vi "Search_1d_array_element.vi"(6 "error in (no error)":errorcluster, 7 "Count in":string[](array[string]), 8 "BD Date":string[](array[string]), 9 "Elements Found in":string[](array[string])) -> (0 "error out":errorcluster, 1 "Count out":string[](array[string]), 3 "Elements Found out":string[](array[string]))   [LabVIEW 2017]
panel:
  out "Table":string[](array[string])
  # "2020-12-03"
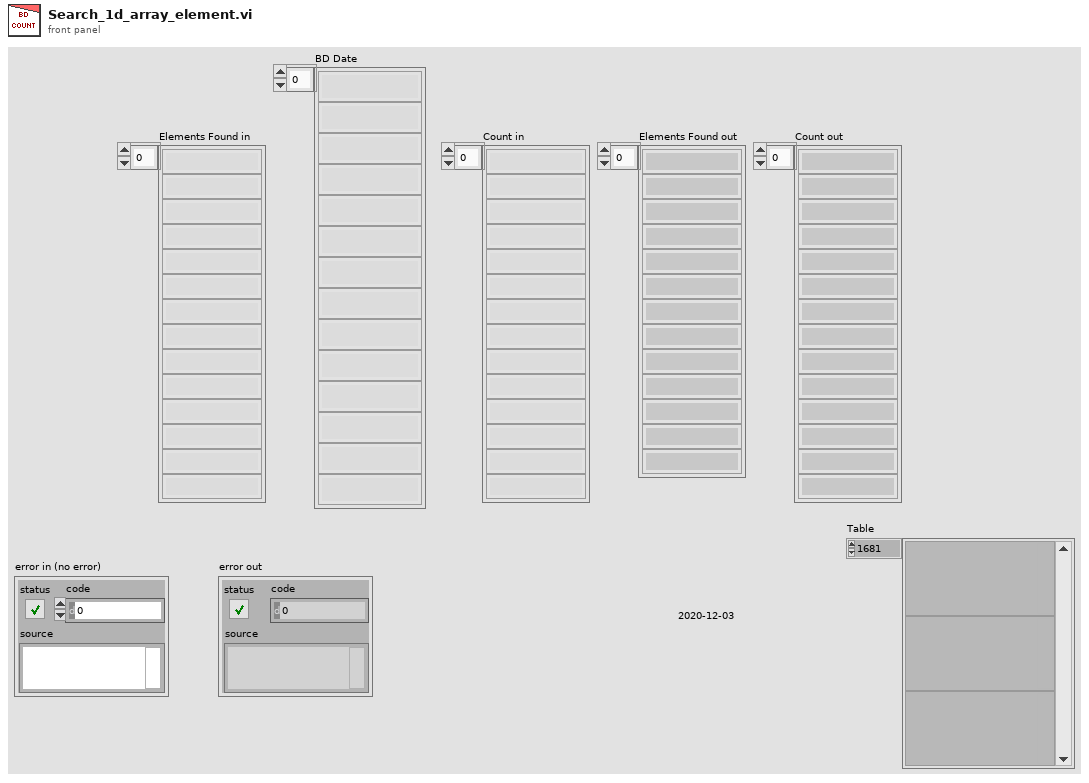
[diagram p1: front panel]
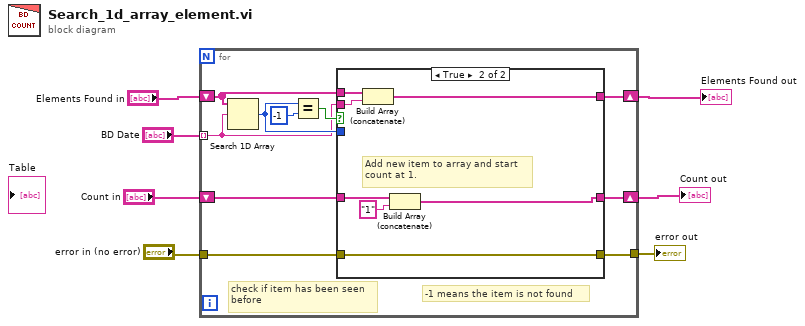
[diagram p0: block diagram]
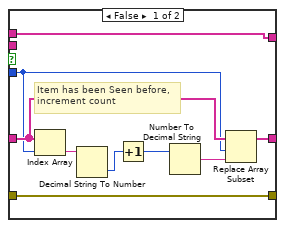
[diagram p2: hidden frame]
diagram:
  n1 = for {
    tunnel: "BD Date" -> [w8] mode=indexing
    shift-right: [w14] -> w7
    shift-left: "Elements Found in" -> [w15]
    shift-right: [w12] -> w1
    shift-left: "Count in" -> [w13]
    tunnel: [w10] -> w3
    tunnel: "error in (no error)" -> [w9]
    # "-1 means the item is not found"
    # "check if item has been seen\nbefore"
    n2 = Search 1D Array(1D array=w15, element=w8) -> (index of element=w11:i32)  [unwired: 1 in]
    n3 = Equal?(x=w11, y=-1) -> (x = y?=w16:bool)
    n4 = case shown="True" w16 {
      tunnel: w15 -> [w26 w33]
      tunnel: [w26 w32] -> w14
      tunnel: w13 -> [w25 w31]
      tunnel: [w23 w30] -> w12
      tunnel: w11 -> [w24 _]
      tunnel: w8 -> [_ w28]
      tunnel: [w18 w27] -> w10
      tunnel: w9 -> [w18 w27]
      frame False {
        # "Item has been Seen before,\nincrement count"
        n5 = Index Array(array=w25, index=w24) -> (element=w22:string)
        n6 = Decimal String To Number(string=w22) -> (number=w21:i32)  [unwired: 2 in, 1 out]
        n7 = Increment(x=w21) -> (x+1=w20:i32)
        n8 = Number To Decimal String(number=w20) -> (decimal integer string=w19:string)  [unwired: 1 in]
        n9 = Replace Array Subset(array=w25, new element=w19, index=w24) -> (w23:string[])
      }
      frame True {
        # "Add new item to array and start\ncount at 1."
        n10 = Build Array (concatenate)(w33, w28) -> (w32:string[])
        n11 = Build Array (concatenate)(w31, "1") -> (w30:string[])
      }
    }
  }
  "Count out" <- w1
  "Elements Found out" <- w7
  "error out" <- w3
